vi "Read IFD Entry.vi"(4 "Directory Offset in":i32, 5 "Image Data in":u8[](array[numeric])) -> (0 "Cluster":T1, 1 "Directory Offset Out":i32, 2 "Image Data Out":u8[](array[numeric]))   [LabVIEW 2012, in "TIFF File Reader.lvlib"]
doc: "Reads the next tag entry in the Image File Directory in a tiff file byte stream, returning the tag, its format and location in the byte stream."
uses:
  TIFF File Reader.lvlib
  IFD Entry.ctl
  FieldTypes.ctl
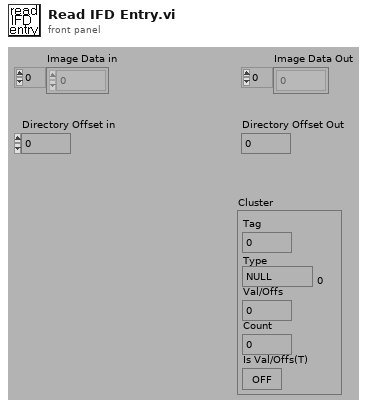
[diagram p1: front panel]
types:
  T1 = typedef "TIFF File Reader.lvlib/IFD Entry.ctl" = cluster{"Tag":u16, "Type":T2, "Count":u32, "Val/Offs":u32, "Is Val/Offs(T)":bool}
  T2 = typedef "TIFF File Reader.lvlib/FieldTypes.ctl" = enum16{"NULL", "U8", "ASCII7", "U16", "U32", "RATIONAL", "SByte(I8)", "Undef(8Bit)", "I16", "I32", "SRat(4B:4B)", "SGL(4Byte)", "DBL(8Byte)"}
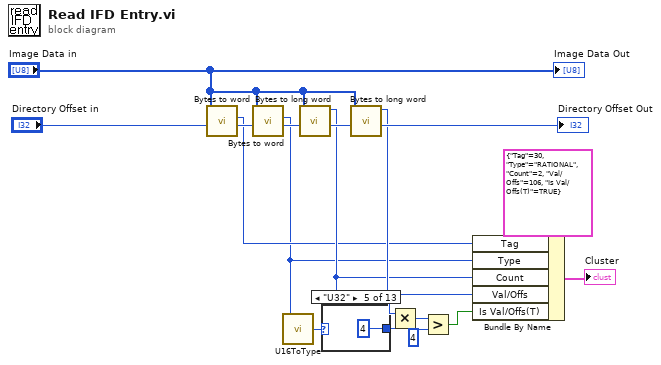
[diagram p0: block diagram]
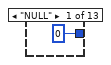
[diagram p2: hidden frame]
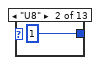
[diagram p3: hidden frame]
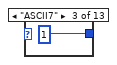
[diagram p4: hidden frame]
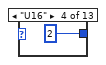
[diagram p5: hidden frame]
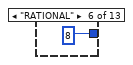
[diagram p6: hidden frame]
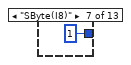
[diagram p7: hidden frame]
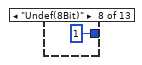
[diagram p8: hidden frame]
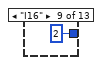
[diagram p9: hidden frame]
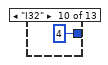
[diagram p10: hidden frame]
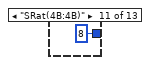
[diagram p11: hidden frame]
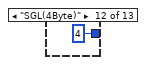
[diagram p12: hidden frame]
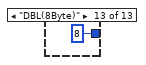
[diagram p13: hidden frame]
diagram:
  n1 = call "Bytes to word.vi"("Index"="Directory Offset in", "Image Data in"="Image Data in") -> ("Index+2"=w14:i32, "Word"=w2:u16)  [unwired: 1 in, 5 out]
  n2 = call "Bytes to word.vi"("Index"=w14, "Image Data in"="Image Data in") -> ("Index+2"=w13:i32, "Word"=w1:u16)  [unwired: 1 in, 5 out]
  n3 = call "U16ToType.vi"("U16 In"=w1) -> ("Type out"=w9:T2)  [unwired: 4 out]
  n4 = call "Bytes to long word.vi"("Index"=w13, "Image Data in"="Image Data in") -> ("Index+4"=w12:i32, "U32"=w7:u32)  [unwired: 6 out]
  n5 = case shown="\"U32\"" w9 {
    tunnel: [i64 0 i64 1 i64 1 i64 2 i64 4 i64 8 i64 1 i64 1 i64 2 i64 4 i64 8 i64 4 i64 8] -> w8
    frame "NULL" {
    }
    frame "U8" {
    }
    frame "ASCII7" {
    }
    frame "U16" {
    }
    frame "U32" {
    }
    frame "RATIONAL" {
    }
    frame "SByte(I8)" {
    }
    frame "Undef(8Bit)" {
    }
    frame "I16" {
    }
    frame "I32" {
    }
    frame "SRat(4B:4B)" {
    }
    frame "SGL(4Byte)" {
    }
    frame "DBL(8Byte)" {
    }
  }
  n6 = call "Bytes to long word.vi"("Index"=w12, "Image Data in"="Image Data in") -> ("Index+4"=→"Directory Offset Out":i32, "U32"=w10:u32)  [unwired: 6 out]
  n7 = Multiply(x=w7, y=w8) -> (x*y=w6:i64)
  n8 = Greater?(x=w6, y=i64 4) -> (0:w4:bool)
  n9 = Bundle By Name(cluster=T1 {"Tag"=30, "Type"=enum."RATIONAL", "Count"=2, "Val/Offs"=106, "Is Val/Offs(T)"=TRUE} ("Cluster"), "Tag"=w2, "Type"=w1, "Count"=w7, "Val/Offs"=w10, "Is Val/Offs(T)"=w4) -> (→"Cluster":T1)
  "Image Data Out" <- "Image Data in"
